vi "Change string.vi"(11 "string":string) -> (3 "String":string)   [LabVIEW 2009]
panel:
  out "unsigned byte array":u8[](array[numeric])
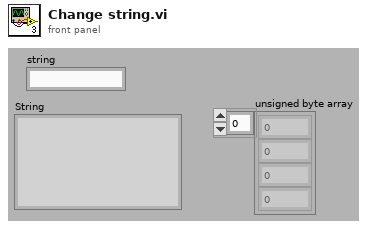
[diagram p1: front panel]
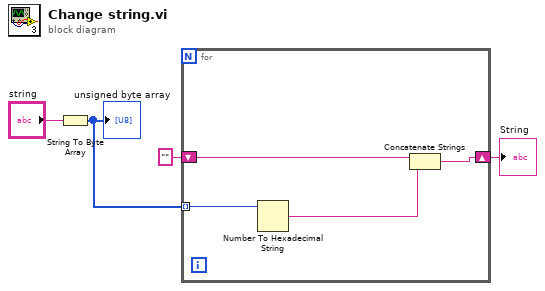
[diagram p0: block diagram]
diagram:
  n1 = String To Byte Array(string="string") -> (unsigned byte array=w4:u8[])
  "unsigned byte array" <- w4
  n2 = for {
    tunnel: w4 -> [w8] mode=indexing
    shift-right: [w5] -> w3
    shift-left: "" -> [w7]
    n3 = Number To Hexadecimal String(2:w8) -> (0:w6:string)  [unwired: 1 out]
    n4 = Concatenate Strings(w7, w6) -> (w5:string)
  }
  "String" <- w3
